vi "Adquirir entre cursores.vi"(8 "error in":errorcluster, 10 "Input Cluster":T1, 11 "WaveformGraph in":refnum<vi>) -> (0 "error out":errorcluster, 2 "Output Cluster":T1)   [LabVIEW 2020]
uses:
  Dados consumidor.ctl
  <vilib>/Waveform/WDTOps.llb/WDT Get Waveform Subset DBL.vi
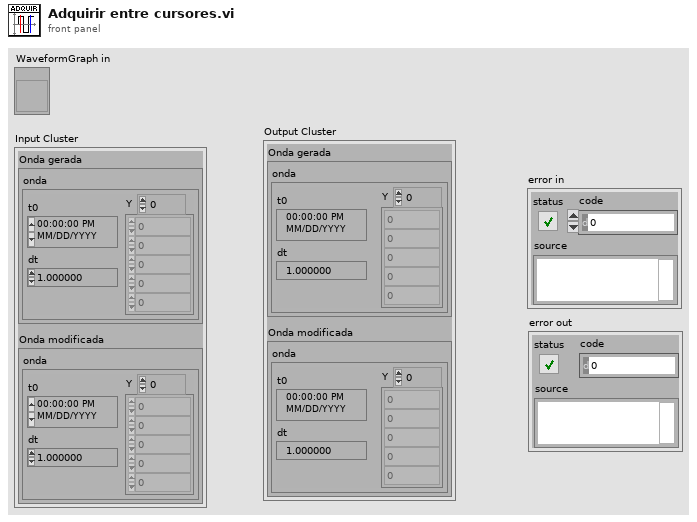
[diagram p1: front panel]
types:
  T1 = typedef "Dados consumidor.ctl" = cluster{"Onda gerada":cluster{"onda":waveform(dbl)}, "Onda modificada":cluster{"onda":waveform(dbl)}}
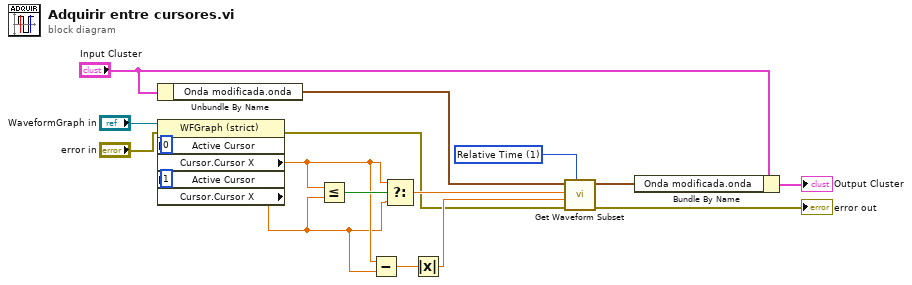
[diagram p0: block diagram]
diagram:
  w16 = u16 1 items=["Samples", "Relative Time"] ("start/duration format")
  n1 = Unbundle By Name("Input Cluster") -> ("Onda modificada.onda"=w15:waveform(dbl))
  n2 = property on="Property Node" class="WFGraph (strict)"(reference="WaveformGraph in", error in="error in", "Active Cursor"=u32 0, "Active Cursor"=u32 1) -> (error out=w3:errorcluster, "Cursor.Cursor X"=w6:dbl, "Cursor.Cursor X"=w5:dbl)  [unwired: 1 out]
  n3 = Less Or Equal?(x=w6, y=w5) -> (x <= y?=w9:bool)
  n4 = Subtract(x=w6, y=w5) -> (x-y=w7:dbl)
  n5 = Select(t=w6, s=w9, f=w5) -> (s? t:f=w8:dbl)
  n6 = Absolute Value(x=w7) -> (abs(x)=w4:dbl)
  n7 = call-poly <vilib>:"Get Waveform Subset.vi"("start/duration format"=w16, "error in (no error)"=w3, "duration"=w4, "start samples/time"=w8, "waveform in"=w15) -> ("error out"=→"error out":errorcluster, "waveform out"=w2:waveform(dbl))  [unwired: 1 in, 2 out]
  n8 = Bundle By Name(cluster="Input Cluster", "Onda modificada.onda"=w2) -> (→"Output Cluster":T1)
